vi "SMTP Email Send File Charset.vi"(0 "recipients":string[](array[string]), 1 "mail server":string, 2 "return address":string, 3 "character set (us-ascii)":string="us-ascii", 5 "subject ([No Subject])":string="[No Subject]", 7 "message":string, 9 "file path":path, 11 "error in (no error)":errorcluster, 12 "binary? (F)":bool, 13 "MIME content-type (application/octet-stream)":string="application/octet-stream", 14 "translit":string="MacRoman iso-8859-1 macroman.trl, ToUpper iso-8859-1 toupper.trl,\nMacRomanUp MacRoman toupper.trl") -> (4 "invalid recipients":string[](array[string]), 15 "error out":errorcluster)   [LabVIEW 2011, in "NewNI_SMTPEmail.lvlib"]
doc: "Sends an email with an attached file to a list of recipients."
uses:
  NewNI_SMTPEmail.lvlib
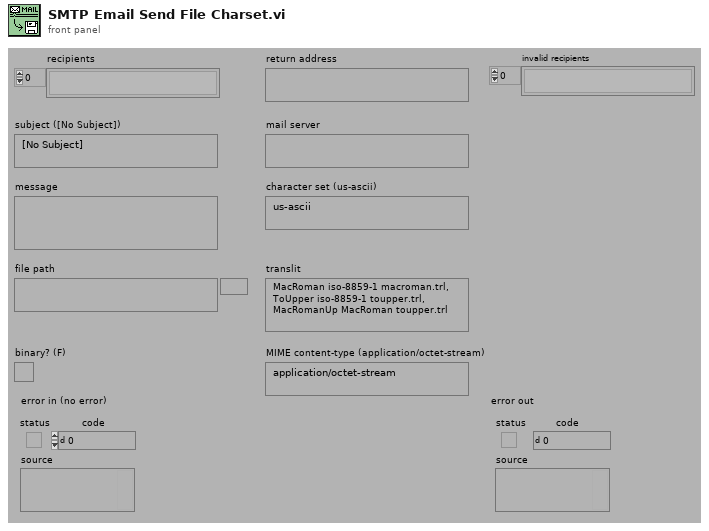
[diagram p1: front panel]
types:
  T1 = typedef "NewNI_SMTPEmail.lvlib/SMTP Email Session.ctl" = refnum<k1>
  T2 = cluster{"file path":path, string, "binary? (F)":bool, "MIME content-type (application/octet-stream)":string}
  T3 = cluster{"file path":path, string, "binary? (F)":bool, "MIME content-type (application/octet-stream)":string}[]
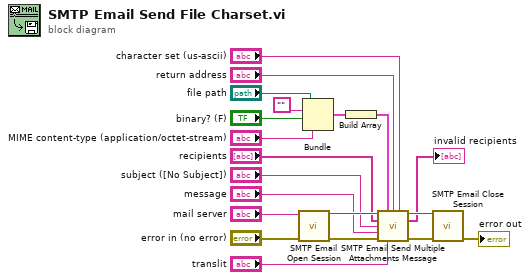
[diagram p0: block diagram]
diagram:
  n1 = call "SMTP Email Open Session.vi"("error in (no error)"="error in (no error)", "mail server"="mail server") -> ("error out"=w15:errorcluster, "smtp session out"=w14:T1)  [unwired: 1 in, 3 out]
  n2 = Bundle("file path"="file path", "", "binary? (F)"="binary? (F)", "MIME content-type (application/octet-stream)"="MIME content-type (application/octet-stream)") -> (w19:T2)  [unwired: 1 out]
  n3 = Build Array(w19) -> (w10:T3)
  n4 = call "SMTP Email Send Multiple Attachments Message.vi"("smtp session"=w14, "attachments"=w10, "return address"="return address", "character set"="character set (us-ascii)", "recipients"="recipients", "subject"="subject ([No Subject])", "message"="message", "error in (no error)"=w15, "translit"="translit") -> ("smtp session out"=w16:T1, "invalid recipients"=→"invalid recipients":string[], "error out"=w13:errorcluster)  [unwired: 4 out]
  n5 = call "SMTP Email Close Session.vi"("error in (no error)"=w13, "smtp session"=w16) -> ("error out"=→"error out":errorcluster)  [unwired: 5 out]
